vi "Write File+ [DBL].vi"(6 "1D array":dbl[](array[numeric]) format="%0.3f", 8 "error in (no error)":errorcluster, 9 "pos offset (bytes:0)":i32, 10 "pos mode (rel. to end:1)":enum16{"start", "end", "current"}(ring)=enum."end", 11 "refnum":refnum<file>) -> (0 "error out":errorcluster, 1 "mark afer write (bytes)":i32, 3 "dup refnum":refnum<file>)   [LabVIEW 2010]
doc: "Writes a 2D or 1D array of single-precision numbers (I16) to a byte stream file at the specified location; the default location is at the end of file. The VI does incoming and internal error checking and does not write if an incoming error occurs.\n\nrefnum is the reference number of the open file.\n\npos mode specifies where the write begins relative to pos offset:\n\n 0: at the beginning of the file plus pos offset.\n\n 1: at the end of the file plus pos offset. This is the default value.\n\n 2: at the current file mark plus pos offset.\n\npos offset specifies in bytes how far from the location specified by pos mode that the operation begins. The default value is 0. Byte units rather than I16 (2 byte) units for flexibility, for example, so that a file can contain a text header written with Write File+ (string) followed by arrays of number written with Write File+ [I16].\n\n2D array contains the single-precision numbers the VI writes to the file if 1D array is not wired or is empty.\n\n1D array contains single-precision numbers the VI writes to the file if this input is not empty.\n\nerror in is a cluster of three elements (error?, code, and source) that describe the upstream error state, that is, the existance of any error preceeding the execution of the VI. The VI executes normally only if no incoming error exists; otherwise it merely passes the error in value to error out. error? is TRUE if an error occurred; the default value is FALSE. code is the error code; the default value is 0. source is in most cases the name of the VI or function that produced the error; the default value is an empty string.\n\ndup refnum is a flow-though parameter with the same value as refnum.\n\nmark after write see above.\n\nerror out is a cluster of three elements (error?, code, and source) that describe the error state following the execution of the VI. If an incoming error does not exist, the VI executes normally and error out describes the VI's error state; if an incoming error exists, error out equals error in."
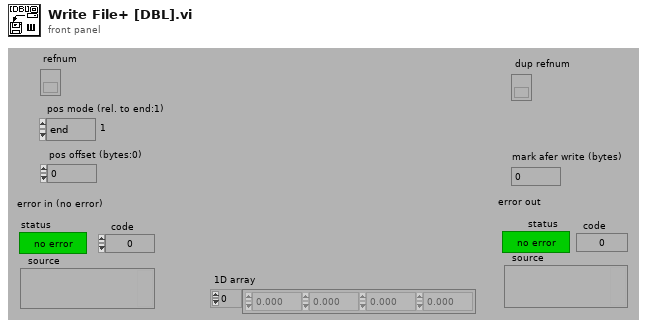
[diagram p1: front panel]
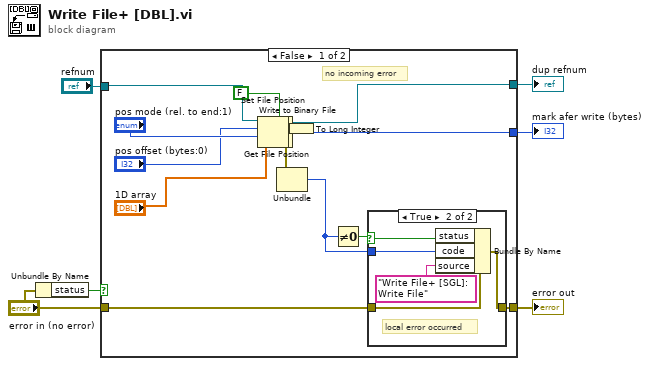
[diagram p0: block diagram]
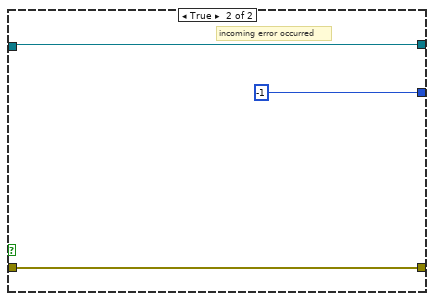
[diagram p3: hidden frame]
diagram:
  n1 = Unbundle By Name("error in (no error)") -> ("status"=w6:bool)
  n2 = case shown="False" w6 {
    tunnel: [w19 w31] -> w5
    tunnel: [w17 -1] -> w2
    tunnel: [w20 w30] -> w4
    tunnel: "refnum" -> [w21 w30]
    tunnel: "error in (no error)" -> [w15 w31]
    frame False {
      # "no incoming error"
      n3 = Set File Position(offset (in bytes) (0)="pos offset (bytes:0)", refnum=w21, from (0:start)="pos mode (rel. to end:1)") -> (refnum out=w12:refnum<file>, error out=w11:errorcluster)  [unwired: 1 in]
      n4 = Write to Binary File(file (use dialog)=w12, data="1D array", error in=w11, 5:FALSE ("prepend array or string size? (T)")) -> (refnum out=w10:refnum<file>, error out=w9:errorcluster)  [unwired: 2 in, 1 out]
      n5 = Get File Position(4:w9, 7:w10) -> (0:w13:errorcluster, 2:w8:i64, 3:w20:refnum<file>)
      n6 = Unbundle(w13) -> ("code"=w16:i32)  [unwired: 2 out]
      n7 = To Long Integer(number=w8) -> (32bit integer=w17:i32)
      n8 = Not Equal To 0?(x=w16) -> (x != 0?=w14:bool)
      n9 = case shown="True" w14 {
        selector: w14 -> [_ w25]
        tunnel: w16 -> [_ w28]
        tunnel: [w24 w29] -> w19
        tunnel: w15 -> [w24 w26]
        frame False {
          # "no local error"
        }
        frame True {
          # "local error occurred"
          n10 = Bundle By Name(cluster=w26, "status"=w25, "code"=w28, "source"="Write File+ [SGL]: Write File") -> (w29:errorcluster)
        }
      }
    }
    frame True {
      # "incoming error occurred"
    }
  }
  "error out" <- w5
  "mark afer write (bytes)" <- w2
  "dup refnum" <- w4
